vi "RunCL - Run All Tests.vi"(11 "Cmd Line Args":string[](array[string])=["C:\\BitBucket\\pipeline_test\\Source\\SampleLV.lvproj", "Main", "My Computer", "1234"]) -> (2 "Error Info":string, 3 "Error Code":i32)   [LabVIEW 2023]
uses:
  <vilib>/addons/_JKI Toolkits/Caraya/classes/Test Report.JUnit/Test Report.JUnit.lvclass
  C:/Program Files (x86)/National Instruments/LabVIEW 2023/vi.lib/addons/_JKI Toolkits/Caraya/classes/Test Report/Test Report.lvclass
  <vilib>/addons/_JKI Toolkits/Caraya/classes/Test Runner.Folder/Test Runner.Folder.lvclass
  C:/Program Files (x86)/National Instruments/LabVIEW 2023/vi.lib/addons/_JKI Toolkits/Caraya/classes/Test Runner/Test Runner.lvclass
  <userlib>/_OpenG.lib/file/file.llb/Append Path to Root if Relative - Scalar__ogtk.vi
  <userlib>/_OpenG.lib/file/file.llb/File Exists - Scalar__ogtk.vi
  <vilib>/addons/_JKI Toolkits/Caraya/classes/Test Runner/Test Runner.lvclass
panel:
  in  "Show Caraya GUI":bool=TRUE
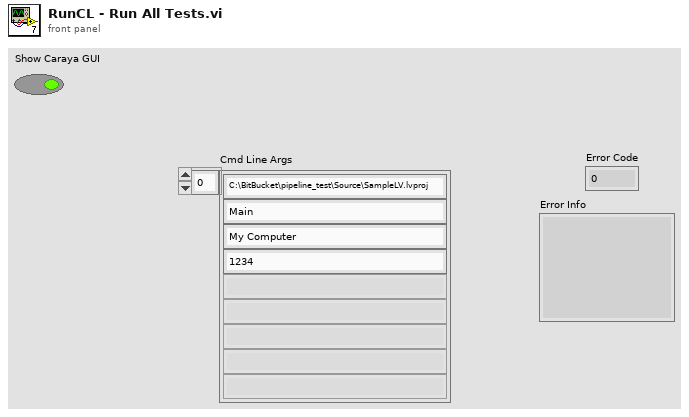
[diagram p1: front panel]
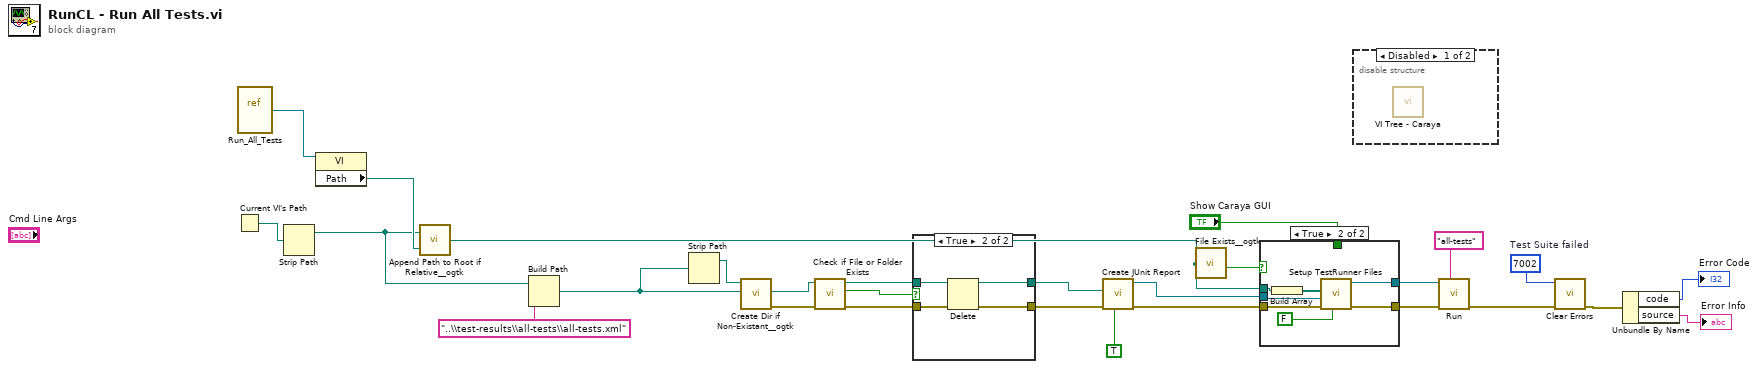
[diagram p0: block diagram]
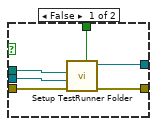
[diagram p3: hidden frame]
diagram:
  w3 = 7002  # Test Suite failed
  n1 = Current VI's Path() -> (path=w26:path)
  n2 = vi-ref "Run_All_Tests.vi"() -> (w27:refnum<vi>)
  n3 = Strip Path(path=w26) -> (stripped path=w6:path)  [unwired: 1 out]
  n4 = property class="VI"(reference=w27) -> ("Path"=w25:path)  [unwired: 1 in, 2 out]
  n5 = call-poly <userlib>:"Append Path to Root if Relative__ogtk.vi"("Absolute or Relative Path"=w25, "Root Path"=w6) -> ("Absolute or Appended Path"=w13:path)
  n6 = Build Path(base path=w6, name or relative path="..\\test-results\\all-tests\\all-tests.xml") -> (appended path=w22:path)
  n7 = Strip Path(path=w22) -> (stripped path=w23:path)  [unwired: 1 out]
  n8 = call <userlib>:"Create Dir if Non-Existant__ogtk.vi"("Directory Path"=w23) -> ("error out"=w9:errorcluster)  [unwired: 8 in, 2 out]
  n9 = call <vilib>:"Check if File or Folder Exists.vi"("error in (no error)"=w9, "path"=w22) -> ("error out"=w8:errorcluster, "file or folder exists?"=w21:bool, "dup path"=w20:path)  [unwired: 7 in]
  n10 = case shown="True" w21 {
    tunnel: w20 -> [w29 w33]
    tunnel: [w29 w32] -> w19
    tunnel: w8 -> [w28 w31]
    tunnel: [w28 w30] -> w7
    frame False {
    }
    frame True {
      n11 = Delete(path (use dialog)=w33, error in=w31) -> (deleted path=w32:path, error out=w30:errorcluster)  [unwired: 3 in, 1 out]
    }
  }
  n12 = call <vilib>:"Create JUnit Report.vi"("Verbose"=TRUE, "error in (no error)"=w7, "Report Path"=w19) -> ("error out"=w10:errorcluster, "Test Report.JUnit out"=w17:refnum<class "Test Report.JUnit.lvclass">)  [unwired: 7 in]
  n13 = call-poly <userlib>:"File Exists__ogtk.vi"("file path"=w13) -> ("exists"=w12:bool)  [unwired: 6 in, 1 out]
  n14 = case shown="True" w12 {
    tunnel: w17 -> [w39 w45]
    tunnel: [w38 w46] -> w16
    tunnel: "Show Caraya GUI" -> [w37 _]
    tunnel: w13 -> [w36 w43]
    tunnel: [w35 w41] -> w11
    tunnel: w10 -> [w34 w40]
    frame False {
      n15 = call <vilib>:"Setup TestRunner Folder.vi"("Interactive (T)"=w37, "error in (no error)"=w34, "Test Report"=w39, "Directory to search"=w36) -> ("error out"=w35:errorcluster, "Test Runner.Folder out"=w38:refnum<class "Test Runner.Folder.lvclass">)  [unwired: 6 in]
    }
    frame True {
      n16 = Build Array(w43) -> (w42:path[])
      n17 = call <vilib>:"Setup TestRunner Files.vi"("Inspect Recursively (T)"=FALSE, "error in (no error)"=w40, "Test Report"=w45, "Paths"=w42) -> ("error out"=w41:errorcluster, "Test Runner.Folder out"=w46:refnum<class "Test Runner.Folder.lvclass">)  [unwired: 6 in]
    }
  }
  n18 = disable-structure shown="Disabled" {
    frame Disabled {
      n19 = call <vilib>:"VI Tree - Caraya.vi"() -> ()  [unwired: 1 in]
    }
    frame Enabled {
    }
  }
  n20 = call <vilib>:"Run.vi"("Name"="all-tests", "error in (no error)"=w11, "Test Runner in"=w16) -> ("error out"=w2:errorcluster)  [unwired: 6 in, 2 out]
  n21 = call <vilib>:"Clear Errors.vi"("error in (no error)"=w2, "specific error code to clear (0: all)"=w3) -> ("error out"=w1:errorcluster)  [unwired: 4 in, 1 out]
  n22 = Unbundle By Name(w1) -> ("code"=→"Error Code":i32, "source"=→"Error Info":string)
